vi "folder_to_string_log_record.vi"(11 "File Path":path) -> (0 "str_fileerrror":string, 1 "str_fileerased":string, 2 "str_filecopyed":string, 3 "str_foldercreat":string)   [LabVIEW 2026]
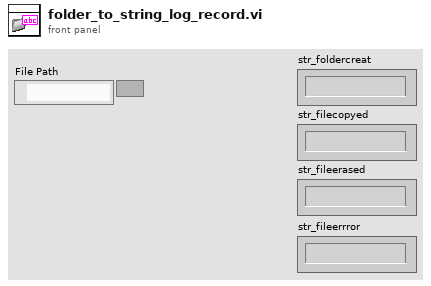
[diagram p1: front panel]
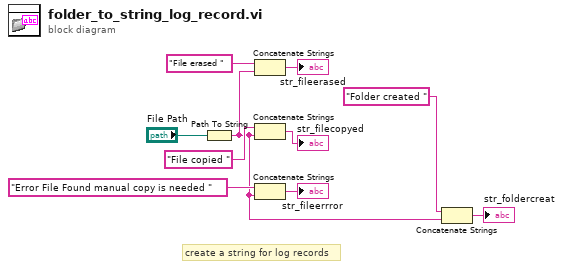
[diagram p0: block diagram]
diagram:
  # "create a string for log records"
  n1 = Path To String(path="File Path") -> (string=w1:string)
  n2 = Concatenate Strings("File erased ", w1) -> (→"str_fileerased":string)
  n3 = Concatenate Strings("File copied ", w1) -> (→"str_filecopyed":string)
  n4 = Concatenate Strings("Error File Found manual copy is needed ", w1) -> (→"str_fileerrror":string)
  n5 = Concatenate Strings("Folder created ", w1) -> (→"str_foldercreat":string)
